vi "Init.vi"(7 "SoL Server":refnum<class "SOL-Server.lvclass">, 8 "error in (no error)":errorcluster) -> (0 "error out":errorcluster, 3 "Approval out":refnum<class "Approval.lvclass">)   [LabVIEW 2020, in "Summer of LabVIEW.lvlib" / "Approval.lvclass"]
uses:
  Approval.lvclass
  Approval.lvclass/Approval.ctl
  SOL-Server/SOL-Server.lvclass
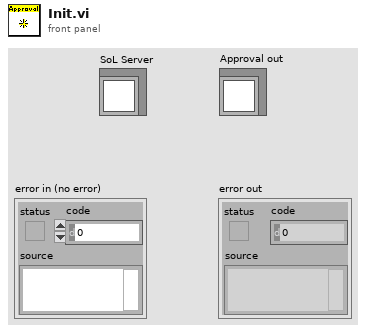
[diagram p1: front panel]
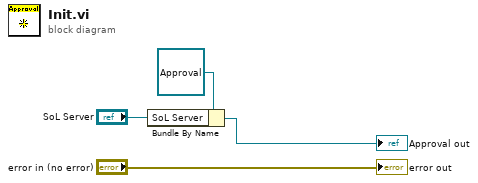
[diagram p0: block diagram]
diagram:
  n1 = Bundle By Name(cluster=refnum<class "Approval.lvclass"> refnum ("Approval in"), "SoL Server"="SoL Server") -> (→"Approval out":refnum<class "Approval.lvclass">)
  "error out" <- "error in (no error)"
